vi "GF_ArmTriggerWave.vi"(1 "error in":errorcluster, 2 "trigger waveform":digitalwaveform[](array[waveform]), 3 "task/channels in":refnum<k21>) -> (0 "error out":errorcluster)   [LabVIEW 2009]
uses:
  <vilib>/DAQmx/write.llb/DAQmx Write (Digital 1D Wfm NChan NSamp).vi
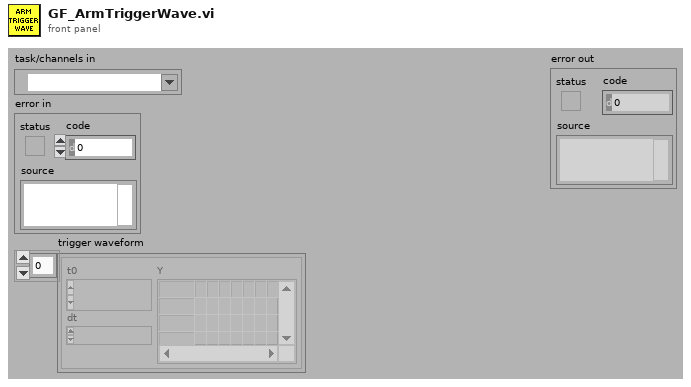
[diagram p1: front panel]
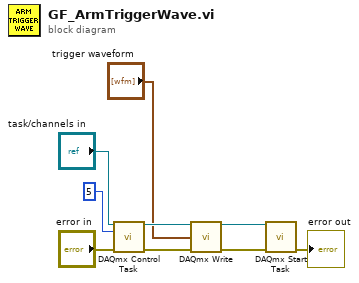
[diagram p0: block diagram]
diagram:
  n1 = call <vilib>:"DAQmx Control Task.vi"("task/channels in"="task/channels in", "action"=5, "error in"="error in") -> ("task out"=w9:refnum<k21>, "error out"=w8:errorcluster)  [unwired: 11 in]
  n2 = call-poly <vilib>:"DAQmx Write.vi"("task/channels in"=w9, "data"="trigger waveform", "error in"=w8) -> ("task out"=w7:refnum<k21>, "error out"=w6:errorcluster)  [unwired: 10 in, 1 out]
  n3 = call <vilib>:"DAQmx Start Task.vi"("task/channels in"=w7, "error in"=w6) -> ("error out"=→"error out":errorcluster)  [unwired: 12 in, 1 out]
